vi "ReadPimentoTXT.vi"() -> ()   [LabVIEW 2022 SP3]
uses:
  <vilib>/Utility/file.llb/Read Delimited Spreadsheet (DBL).vi
panel:
  out "Phase":cluster{"Array":dbl[], "Array":dbl[]}(graph) caption="Amplitude [Hz]"
  in  "Skip First N Lines":i32=48
  out "Magnitude":cluster{"Array":dbl[], "Array":dbl[]}(graph) caption="Amplitude [Hz]"
  out "number of rows":i32
  in  "name or relative path":path=path "C:/Users/LAV-UFSC/OneDrive - UFSC/Documents/LAV - TCC/Dados-Experimentos/25-04/frf_3.txt"
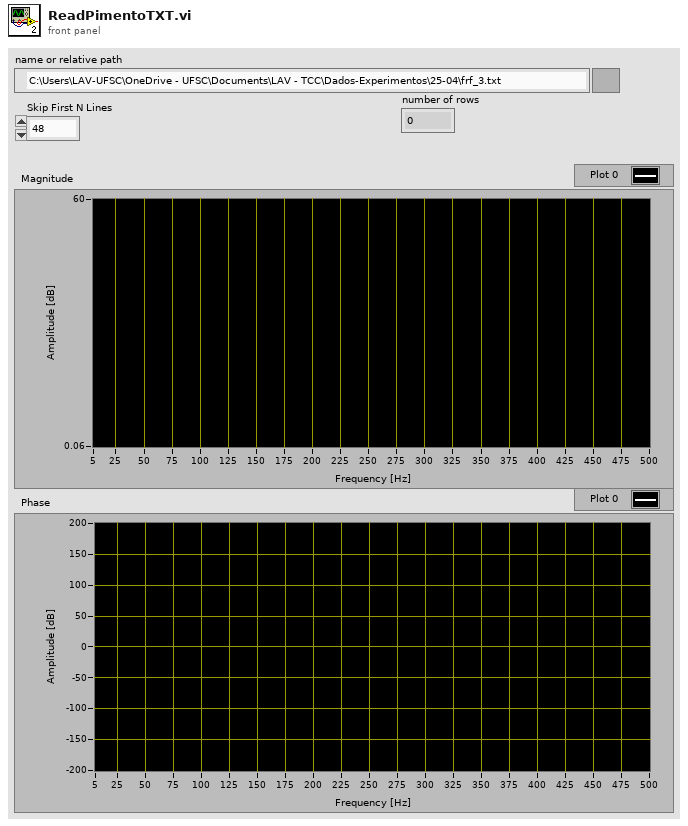
[diagram p1: front panel]
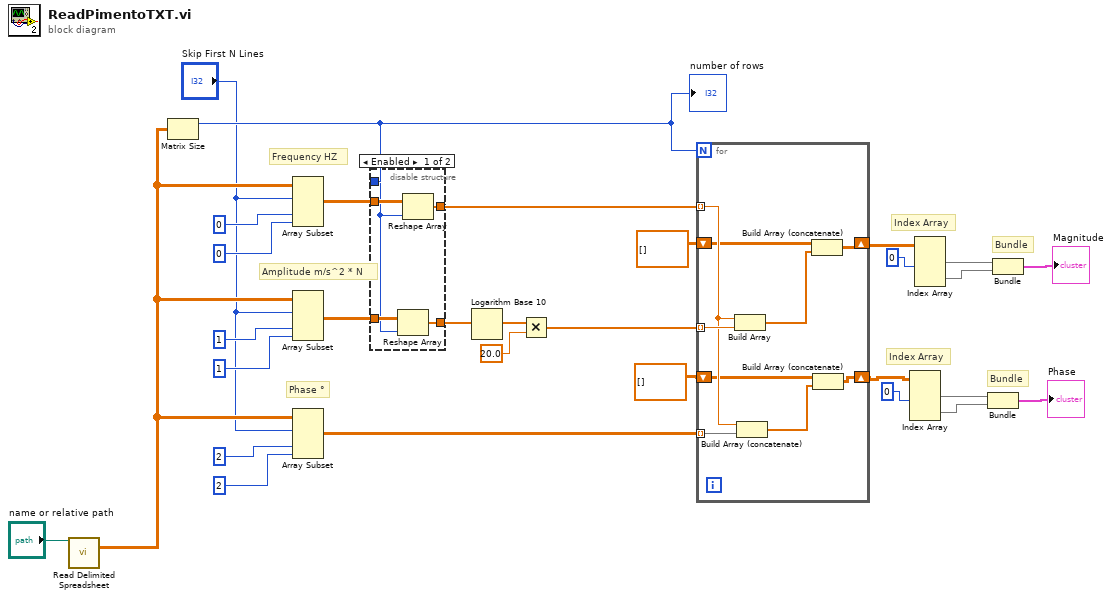
[diagram p0: block diagram]
diagram:
  # "Index Array"
  # "Bundle"
  # "Index Array"
  # "Bundle"
  # "Phase °"
  # "Amplitude m/s^2 * N"
  # "Frequency HZ"
  n1 = call-poly <vilib>:"Read Delimited Spreadsheet.vi"("file path (dialog if empty)"="name or relative path") -> ("all rows"=w19:dbl[][])  [unwired: 9 in, 5 out]
  n2 = Matrix Size(0:w19) -> (1:w18:i32)  [unwired: 1 out]
  "number of rows" <- w18
  n3 = Array Subset(array=w19, index (row)="Skip First N Lines", index (col)=0 ("column 1"), length (col)=0 ("column N")) -> (w23:dbl[][])  [unwired: 1 in]
  n4 = Array Subset(array=w19, index (row)="Skip First N Lines", index (col)=1 ("column 1"), length (col)=1 ("column N")) -> (w22:dbl[][])  [unwired: 1 in]
  n5 = Array Subset(array=w19, index (row)="Skip First N Lines", index (col)=2 ("column 1"), length (col)=2 ("column N")) -> (w21:dbl[][])  [unwired: 1 in]
  n6 = disable-structure shown="Enabled" {
    disable-tunnel: w23 -> [w35 w37]
    disable-tunnel: w22 -> [w34 w36]
    disable-tunnel: [w33 w37] -> w20
    disable-tunnel: [w32 w36] -> w8
    disable-tunnel: w18 -> [w31 _]
    frame Enabled {
      n7 = Reshape Array(w34, w31) -> (w32:dbl[])
      n8 = Reshape Array(w35, w31) -> (w33:dbl[])
    }
    frame Disabled {
    }
  }
  n9 = Logarithm Base 10(1:w8) -> (0:w9:dbl[])
  n10 = Multiply(x=w9, y=20.0) -> (x*y=w7:dbl[])
  n11 = for {
    N: w18 -> [_]
    tunnel: w20 -> [w44] mode=indexing
    tunnel: w7 -> [w45] mode=indexing
    tunnel: w21 -> [w46] mode=indexing
    shift-right: [w41] -> w12
    shift-left: dbl[][] [] -> [w43]
    shift-right: [w40] -> w1
    shift-left: dbl[][] [] -> [w39]
    n12 = Build Array(w44, w45) -> (w42:dbl[])
    n13 = Build Array (concatenate)(w44, w46) -> (w38:dbl[])
    n14 = Build Array (concatenate)(w43, w42) -> (w41:dbl[][])
    n15 = Build Array (concatenate)(w39, w38) -> (w40:dbl[][])
  }
  n16 = Index Array(array=w1, index (col) #1=0 ("disabled index (col)")) -> (element #1=w3:dbl[], element #2=w4:dbl[])  [unwired: 3 in]
  n17 = Index Array(array=w12, index (col) #1=0 ("disabled index (col)")) -> (element #1=w14:dbl[], element #2=w15:dbl[])  [unwired: 3 in]
  n18 = Bundle(w3, w4) -> (→"Phase":cluster{dbl[], dbl[]})  [unwired: 1 in]
  n19 = Bundle(w14, w15) -> (→"Magnitude":cluster{dbl[], dbl[]})  [unwired: 1 in]
